vi "PV ActiveLine - DisplayControlBacklight.vi"(7 "W/R":bool, 8 "Fehler (Eingang)":errorcluster, 9 "Backlight Intensity":u8 max=100 step=1, 11 "Referenz in":refnum<visa-resource-name>) -> (0 "Cluster (Ausgang)":errorcluster, 1 "Backlight Intensity out":u8 max=100 step=1, 3 "Referenz out":refnum<visa-resource-name>)   [LabVIEW 2013, in "PV ActiveLine.lvlib"]
doc: "BAL - Backlight\n\nTransmit: BAL [,a]\nReceive: a\n\nBacklight in percent, a = 0 … 100\n100% is full brightness"
uses:
  <instrlib>/PV ActiveLine/PV ActiveLine.lvlib
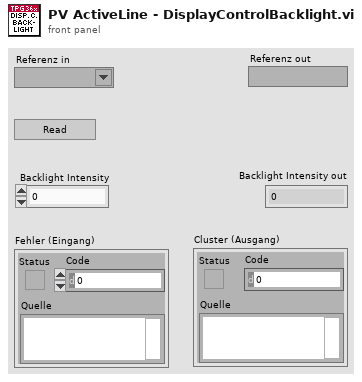
[diagram p1: front panel]
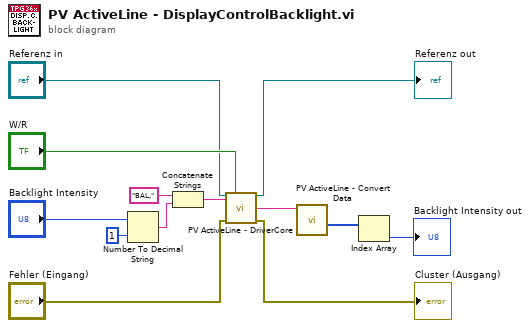
[diagram p0: block diagram]
diagram:
  n1 = Number To Decimal String(number="Backlight Intensity", width (-)=i16 1 ("Breite (-)")) -> (decimal integer string=w9:string)
  n2 = Concatenate Strings("BAL,", w9) -> (w11:string)
  n3 = call <instrlib>:"PV ActiveLine - DriverCore.vi"("Referenz in"="Referenz in", "Write/Read"="W/R", "Command"=w11, "Fehler (Eingang)"="Fehler (Eingang)") -> ("Referenz out"=→"Referenz out":refnum<visa-resource-name>, "String Out"=w5:string, "Cluster (Ausgang)"=→"Cluster (Ausgang)":errorcluster)  [unwired: 9 in]
  n4 = call <instrlib>:"PV ActiveLine - Convert Data.vi"("String in"=w5) -> ("Integer Out"=w4:i32[])  [unwired: 7 in, 3 out]
  n5 = Index Array(array=w4) -> (element=→"Backlight Intensity out":i32)  [unwired: 1 in]
